vi "Poll.vi"(8 "error in (no error)":errorcluster, 10 "Period in ms":u32, 11 "Zero Timeout Message Handler in":refnum<class "Zero Timeout Message Handler.lvclass">) -> (0 "error out":errorcluster, 3 "Zero Timeout Message Handler out":refnum<class "Zero Timeout Message Handler.lvclass">)   [LabVIEW 2024, in "Zero Timeout Message Handler.lvlib" / "Zero Timeout Message Handler.lvclass"]
uses:
  Zero Timeout Message Handler.lvclass
  <vilib>/addons/control/pid/pid.llb/PID (DBL).vi
  Zero Timeout Message Handler.lvclass/Zero Timeout Message Handler.ctl
  <vilib>/addons/control/pid/NI_PID_pid.lvlib
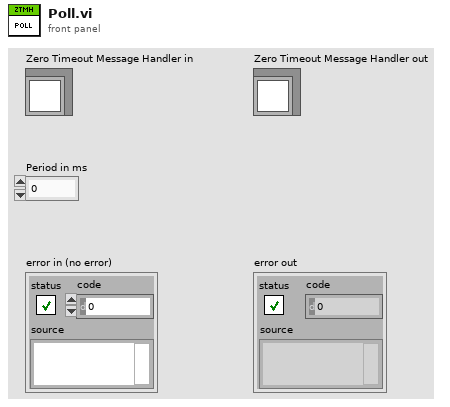
[diagram p1: front panel]
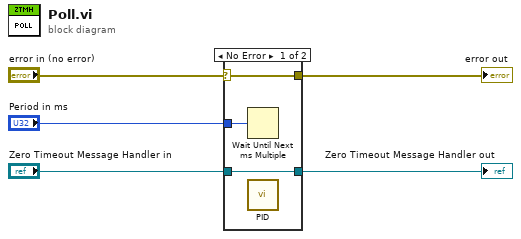
[diagram p0: block diagram]
diagram:
  n1 = case shown="No Error" "error in (no error)" {
    selector: "error in (no error)" -> [w8 w10]
    tunnel: [w8 w10] -> w4
    tunnel: [w7 w9] -> w2
    tunnel: "Zero Timeout Message Handler in" -> [w7 w9]
    tunnel: "Period in ms" -> [w6 _]
    frame No Error {
      n2 = Wait Until Next ms Multiple(millisecond multiple=w6) -> ()  [unwired: 1 out]
      n3 = call-poly <vilib>:"PID.vi"() -> ()  [unwired: 10 in, 2 out]
    }
    frame Error {
    }
  }
  "error out" <- w4
  "Zero Timeout Message Handler out" <- w2
